vi "lvGetInstalledNISoftware.vi"   [LabVIEW 2015]
uses:
  <vilib>/nisyscfg/nisyscfg.lvlib
  <vilib>/nisyscfg/Get Installed Components.vi
  <vilib>/nisyscfg/Component Types.ctl
  <vilib>/nisyscfg/Close (System).vi
types:
  T1 = enum16{"open", "replace", "create", "open or create", "replace or create", "replace or create with confirmation"}
  T2 = typedef "nisyscfg.lvlib/Component Types.ctl" = u32
  T3 = typedef "nisyscfg.lvlib/Software 1.2.ctl" = cluster{"title":string, "description":string, "ID":string, "version":string, "component type":T4}
  T4 = typedef "nisyscfg.lvlib/Component Type.ctl" = u32
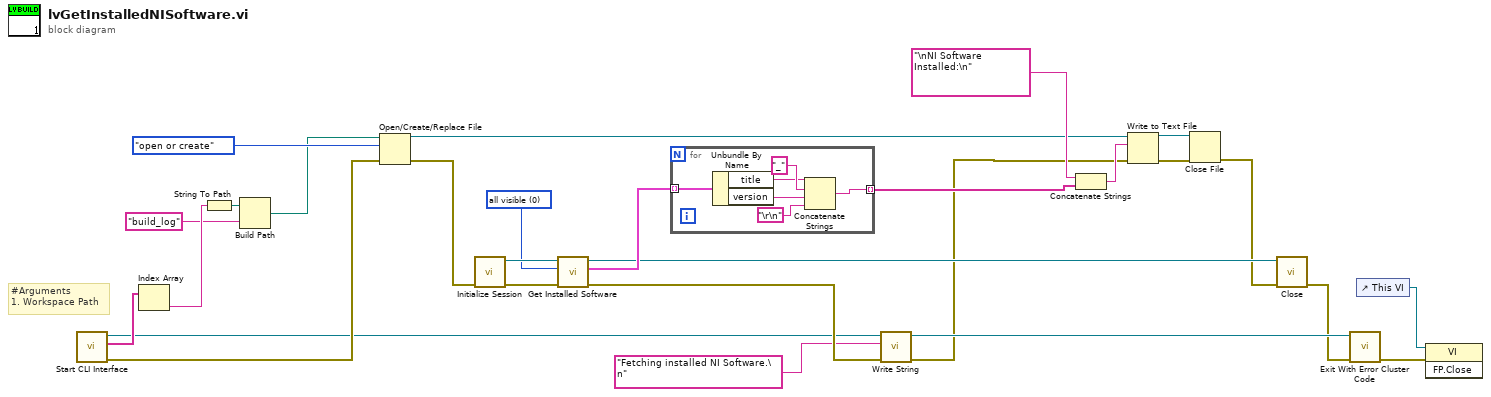
[diagram p0: block diagram]
diagram:
  w26 = T2 0 items=["all visible", "all including hidden", "standard only", "startup only"] ("Item Types (all visible)")
  # "#Arguments\n1. Workspace Path"
  n1 = call <vilib>:"Start CLI Interface.vi"() -> ("error out"=w18:errorcluster, "Custom Parameters"=w21:string[], "CLI out"=w16:refnum<class "CLI.lvclass">)  [unwired: 9 in]
  n2 = Index Array(array=w21) -> (element=w20:string)  [unwired: 1 in]
  n3 = String To Path(string=w20) -> (path=w8:path)
  n4 = Build Path(base path=w8, name or relative path="build_log") -> (appended path=w6:path)
  n5 = Open/Create/Replace File(file path (use dialog)=w6, error in=w18, operation (0:open)=T1."open or create") -> (refnum out=w1:refnum<file>, error out=w7:errorcluster)  [unwired: 3 in, 1 out]
  n6 = call <vilib>:"Initialize Session.vi"("error in (no error)"=w7) -> ("error out"=w28:errorcluster, "Session out"=w27:refnum<k21>)  [unwired: 9 in]
  n7 = call-poly <vilib>:"Get Installed Software.vi"("error in (no error)"=w28, "Item Types (all visible)"=w26, "Session in"=w27) -> ("error out"=w17:errorcluster, "Software Components"=w25:T3[], "Session out"=w24:refnum<k21>)  [unwired: 6 in]
  n8 = for {
    tunnel: w25 -> [w34] mode=indexing
    tunnel: [w30] -> w10 mode=indexing
    n9 = Unbundle By Name(w34) -> ("title"=w32:string, "version"=w31:string)
    n10 = Concatenate Strings(w32, "_" ("string"), w31, "\r\n") -> (w30:string)
  }
  n11 = call <vilib>:"Write String.vi"("error in (no error)"=w17, "Text to Write"="Fetching installed NI Software.\n", "CLI in"=w16) -> ("error out"=w2:errorcluster, "CLI out"=w14:refnum<class "CLI.lvclass">)  [unwired: 7 in]
  n12 = Concatenate Strings("\nNI Software Installed:\n" ("string"), w10) -> (w3:string)
  n13 = Write to Text File(file (use dialog)=w1, text=w3, error in=w2) -> (refnum out=w4:refnum<file>, error out=w5:errorcluster)  [unwired: 1 in, 1 out]
  n14 = Close File(refnum=w4, error in=w5) -> (error out=w22:errorcluster)  [unwired: 1 out]
  n15 = call-poly <vilib>:"Close.vi"("error in (no error)"=w22, "Session in"=w24) -> ("error out"=w13:errorcluster)  [unwired: 9 in]
  n16 = call <vilib>:"Exit With Error Cluster Code.vi"("error in (no error)"=w13, "CLI in"=w14) -> ("error out"=w12:errorcluster)  [unwired: 9 in]
  n17 = control-ref of="This VI"() -> (w11:refnum<vi>)
  n18 = invoke class="VI" method="FP.Close"(reference=w11, error in=w12) -> ()  [unwired: 1 in, 3 out]
